vi "Dashboard Main.vi"() -> ()   [LabVIEW 2017]
uses:
  <vilib>/Utility/miscctls.llb/LVRowAndColumnTypeDef.ctl
  <vilib>/event_ctls.llb/eventvkey.ctl
  <vilib>/Rock Robotics/Network Tables/NT Read Numeric Array.vi
  <vilib>/Rock Robotics/Network Tables/NT Read Boolean.vi
  <vilib>/Rock Robotics/WPI/Dashboard/WPI_DashboardLogging Global.vi
panel:
  in  "Camera Settings Right":T1={"Frame Rate"=30, "Compression"=30, "Size"=1, "DB Camera Config"=FALSE} {"Frame Rate" scale=1.0..30.0; "Compression" scale=100.0..-1.0; "Size" items=["640x480", "320x240", "160x120"]}
  in  "Camera Name Right":string(combo)="No Camera Selection"
  out "Camera Info":cluster{"Mbps LED":bool, "Mbps":dbl, "fps":dbl} {"fps" format="%#.1g"; "Mbps" format="%#.1g"}
  in  "Camera Settings":T1={"Frame Rate"=30, "Compression"=30, "Size"=1, "DB Camera Config"=FALSE} {"Frame Rate" scale=1.0..30.0; "Compression" scale=100.0..-1.0; "Size" items=["640x480", "320x240", "160x120"]}
  in  "TCP":refnum<k5>
  in  "Rec Mode":enum32{"Stop", "Record", "Playback"}(radio)
  out "Robot IP":string
  out "Image Message":string="Timeout in Camera Communications"
  in  "Dashboard Tab":T2(tab)
  out "?":bool
  out "?":bool
  out "?":dbl
  in  "Select Auto":string(combo)="Select Autonomous ..."
  out "NT Connection":bool
  out "MotorChart R":cluster{"Numeric":dbl, "Numeric":dbl}(graph)
  out "MotorChart L":cluster{"Numeric":dbl, "Numeric":dbl}(graph)
  out "MotorSliders R":cluster{"MotorSlide1":dbl, "MotorSlide2":dbl} {"MotorSlide2" scale=-1.0..1.0 scale format="%#_2e"; "MotorSlide1" scale=-1.0..1.0 scale format="%#_2e"}
  out "MotorSliders L":cluster{"MotorSlide1":dbl, "MotorSlide2":dbl} {"MotorSlide2" scale=-1.0..1.0 scale format="%#_2e"; "MotorSlide1" scale=-1.0..1.0 scale format="%#_2e"}
  out "Gyro":dbl(knob) scale=0.0..360.0
  out "JS1 Z":dbl(slide) scale=-1.0..1.0 scale format="%#_2e"
  out "JS1 Graph":cluster{"X":dbl, "Y":dbl}[](graph)
  out "JS1 Buttons":T3
  out "JS2 Z":dbl(slide) scale=-1.0..1.0 scale format="%#_2e"
  out "JS2 Graph":cluster{"X":dbl, "Y":dbl}[](graph)
  out "JS2 Buttons":T3
  out "Mode":T4(ring)=enum."Auto Disabled"
  out "Camera Image Right":T5(plugin-control)
  in  "DB/String 9":string
  in  "DB/String 8":string
  in  "DB/String 7":string
  in  "DB/String 6":string
  in  "DB/String 5":string
  in  "DB/String 4":string
  in  "DB/String 3":string
  in  "DB/String 2":string
  in  "DB/String 1":string
  in  "DB/String 0":string
  in  "DB/Slider 0":dbl(slide) scale=0.0..5.0
  in  "DB/Slider 1":dbl(slide) scale=0.0..5.0
  in  "DB/Slider 2":dbl(slide) scale=0.0..5.0
  in  "DB/Slider 3":dbl(slide) scale=0.0..5.0
  out "DB/LED 3":bool
  out "DB/LED 2":bool
  out "DB/LED 1":bool
  out "DB/LED 0":bool
  in  "DB/Button 3":bool
  in  "DB/Button 2":bool
  in  "DB/Button 1":bool
  in  "DB/Button 0":bool caption="New Name"
  in  "Test Slider":dbl(slide) scale=0.0..100.0 scale format="%#_3g"
  in  "On/Off":bool caption="Solenoid"
  in  "Test Name":u16(ring) items=["Select the test to run..."]
  in  "Test Tree":string(tree)
  in  "Motor":cluster{"Value":dbl, "Enable":bool} {"Value" scale=-1.0..1.0 scale format="%#_3g"}
  out "Progress":T6 {"Test Progress" scale=0.0..100.0}
  in  "Rev/Fwd":cluster{"Forward":bool, "Reverse":bool}
  in  "Test Ring":u16(ring) items=["Monochrome", "Color"]
  out "Cmd Status":string
  in  "Execute Command":bool
  in  "Command Params":string[][](table)
  in  "Command Selection":i32(listbox)
  in  "CheckList":i32(listbox)
  out "Tree":string(tree)
  out "Camera Image":T5(plugin-control)
  out "Background":bool
  in  "Camera Name":string(combo)="No Camera Selection"
  # "HW"
  # "HW"
  # "Joysticks"
  # "Ultrasonic Distance"
  # "Drive Motors"
  # "Front"
  # "Limit Switch Position"
  # "Compressor On/Off"
  # "Right"
  # "Left"
  # "Back"
  # "This tab is a great place for autonomous settings and robot-specific values.\nPlace controls and indicators inside this tab and match name to\nDashboard Variables on robot. You can also delete this comment."
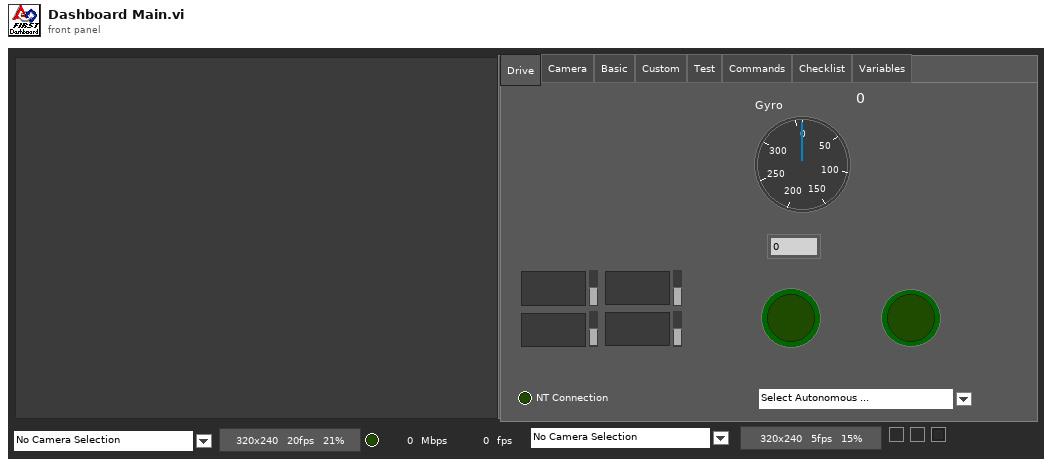
[diagram p1: front panel]
types:
  T1 = cluster{"Frame Rate":i32, "Compression":i32, "Size":u16, "DB Camera Config":bool}
  T2 = enum32{"Drive", "Camera", "Basic", "Custom", "Test", "Commands", "Checklist", "Variables"}
  T3 = cluster{bool, bool, bool, bool, bool, bool, bool, bool, bool, bool, bool, bool}
  T4 = enum8{"Tele-Op Disabled", "Tele-Op Enabled", "Auto Disabled", "Auto Enabled", "Test Disabled", "Test Enabled", "Disconnected", "No Code", "E-Stop"}
  T5 = typedef "IMAQ Image.ctl" = refnum<image>
  T6 = cluster{"Test Progress":u8, "Test Progress Text":string}
  T7 = cluster{"Save Path":path, "Interval (s)":dbl, "Keep":i32}
  T8 = typedef "Image Type" = u32
  T9 = cluster{"IDs":cluster{"RPC field ID":u16, "Unique ID":u16}, "String":string}
  T10 = cluster{"Error Strings":string, "Disable Counts":cluster{u16, u16}, "Rail Faults":cluster{u16, u16, u16}, "Robot IP":string, "DB Mode":u8, "Event Info":cluster{"Name":string, "Type":u8, "Number":u16, "Replay":u8}}
  T11 = cluster{"Storage":cluster{"Disk Free":u64, "RAM Block":u32, "RAM free":u32}, "CPU Utilization":cluster{"CPU % ISR":sgl, "CPU % Time Crit":sgl, "CPU % Timed Str":sgl, "CPU % High":sgl, "CPU % Above":sgl, "CPU % Normal":sgl, "CPU % Low":sgl}, "CAN":cluster{"% Bus Utilization":sgl, "Bus Off Cnt":u32, "TX_FIFO Full Cnt":u32, "Receive Error Cnt":u8, "Transmit Error Cnt":u8}, "HID":cluster{"HID Outputs":u32, "Rumble Low":u16, "Rumble High":u16}[]}
  T12 = cluster{"Status bits":cluster{"Test Mode":bool, "Autonomous":bool, "Enabled":bool, "Code Start":bool, "Brownout":bool, "Reserved 2":bool, "Reserved 3":bool, "E-Stop":bool}, "Code Trace":cluster{"Disabled":bool, "TeleOp":bool, "Auto":bool, "Test":bool}, "Controller Type":enum16{"unknown", "cRIO", "roboRio"}, "Code?":enum16{"unknown", "noCode", "code"}, "Battery V":dbl}
  T13 = cluster{"Control Bits":cluster{"TestMode":bool, "Autonomous":bool, "Enabled":bool, "FMS Present":bool, bool, bool, bool, "E-Stop":bool}, "Team Station ":u8, "Countdown":sgl, "Joystick Values":cluster{"Axes":dbl[], "Buttons":bool[], "POVs":i16[]}[]}
  T14 = cluster{"Axes":dbl[], "Buttons":bool[], "POVs":i16[]}[]
  T15 = cluster{"Axes":dbl[], "Buttons":bool[], "POVs":i16[]}
  T16 = cluster{"Buttons[0]":bool, "Buttons[1]":bool, "Buttons[2]":bool, "Buttons[3]":bool, "Buttons[4]":bool, "Buttons[5]":bool, "Buttons[6]":bool, "Buttons[7]":bool, "Buttons[8]":bool, "Buttons[9]":bool, "Buttons[10]":bool, "Buttons[11]":bool}
  T17 = cluster{"Camera Image":refnum<vi>, "Dashboard Tab":refnum<vi>, "Background":refnum<vi>, "Rec Mode":refnum<vi>, "Test Slider":refnum<vi>, "On/Off ":refnum<vi>, "Test Ring":refnum<vi>, "Rev/Fwd":refnum<vi>, "Test Name":refnum<vi>, "Motor":refnum<vi>, "Progress":refnum<vi>, "CheckList":refnum<vi>, "Tree":refnum<vi>, "Test Tree":refnum<vi>, "Command Params":refnum<vi>, "Command Selection":refnum<vi>, "Execute Command":refnum<vi>, "Cmd Status":refnum<vi>, "Camera Settings":refnum<vi>, "Camera Name":refnum<vi>, "Camera Info":refnum<vi>, "Camera Settings Right":refnum<vi>, "Camera Name Right":refnum<vi>, "Camera Image Right":refnum<vi>}
  T18 = cluster{"Camera Name":string, string, "Saved DB Images Info":cluster{"Save Path":path, "Interval (s)":dbl, "Keep":i32}}
  T19 = cluster{"Camera Name Right":string, string, "Saved DB Images Info":cluster{"Save Path":path, "Interval (s)":dbl, "Keep":i32}}
  T20 = cluster{"Operation":enum16{"Update", "Clear"}, "Color Box":u32}[]
  T21 = typedef "eventvkey.ctl" = enum16{"ASCII", "Enter", "Return", "Shift", "Ctrl", "Alt", "Cmd", "Opt", "Caps", "NumLock", "Clear", "Break", "Up", "Down", "Left", "Right", "Insert", "Delete", "Home", "End", "PageUp", "PageDown", "Escape", "Help", "Pause", "ScrollLock", "F1", "F2", "F3", "F4", "F5", "F6", "F7", "F8", "F9", "F10", "F11", "F12", "F13", "F14", "F15", "F16", "F17", "F18", "F19", "F20", "F21", "F22", "F23", "F24", "Play", "VolumeUp", "VolumeDown", "Mute", "Two Byte Char"}
  T22 = cluster{"Image Size":bool, "Image Type":bool, "Pixel Value":bool, "ROI Information":bool, "Zoom Factor":bool}
  T23 = cluster{"Operation":enum16{"Update", "Clear"}, "Color Box":u32}
  T24 = typedef "LVRowAndColumnTypeDef.ctl" = cluster{"Row":i32, "Column":i32}
  T25 = cluster{"Shift":bool, "Ctrl":bool, "Alt":bool, "Cmd":bool, "Opt":bool}
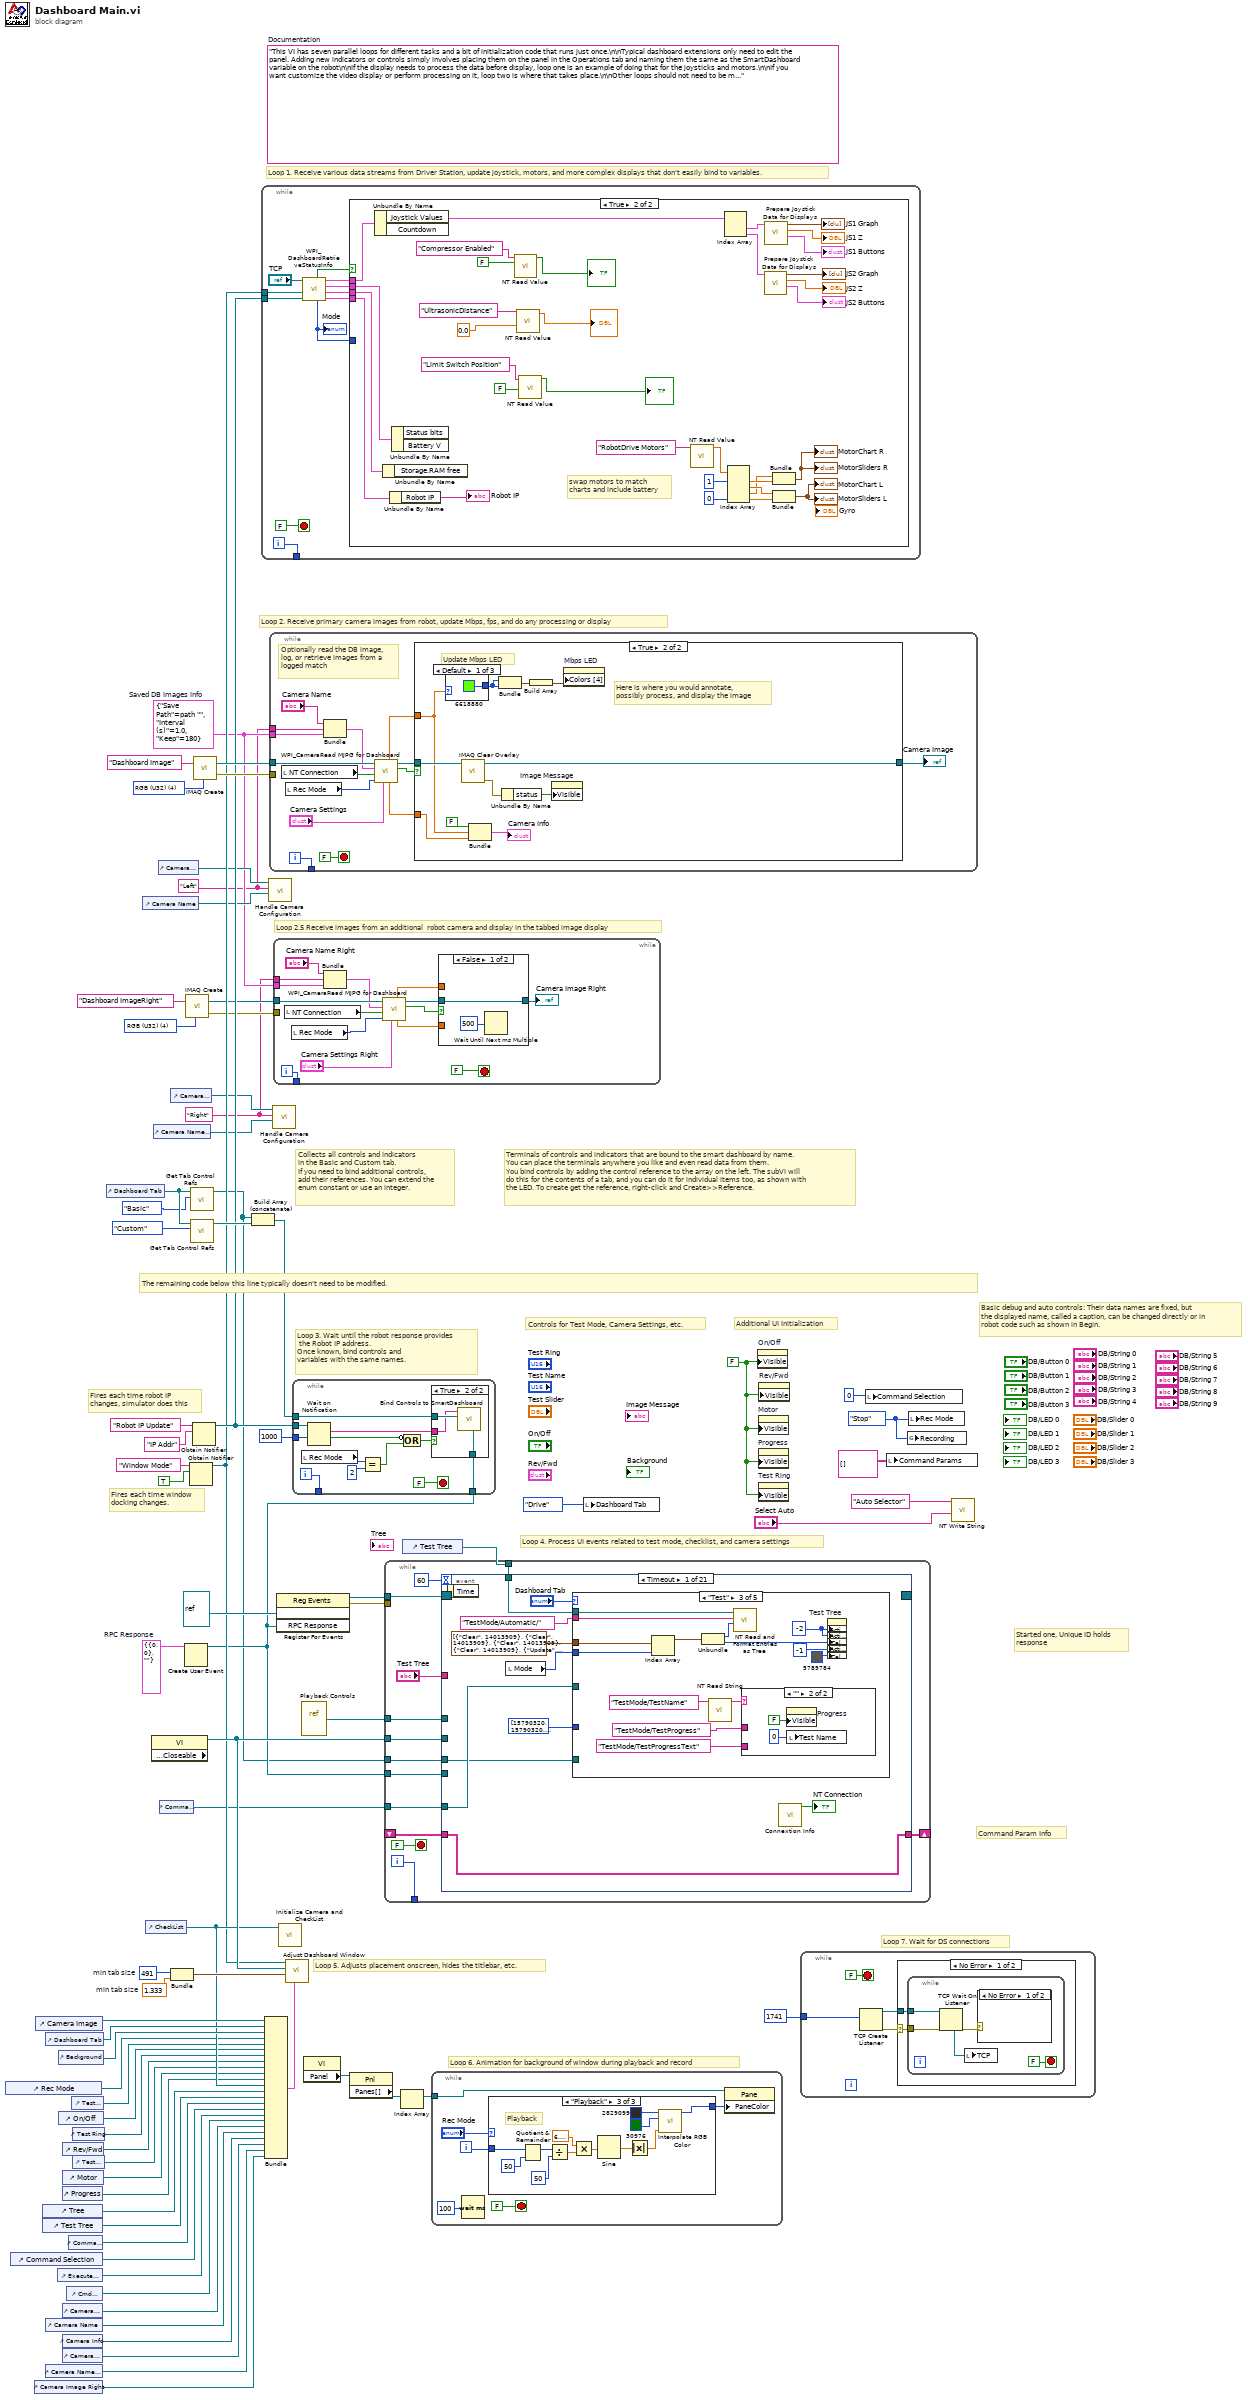
[diagram p0: block diagram]
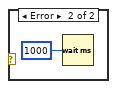
[diagram p3: hidden frame]
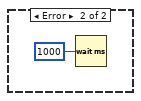
[diagram p4: hidden frame]
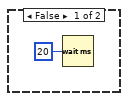
[diagram p5: hidden frame]
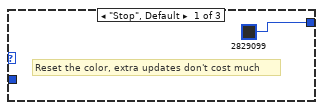
[diagram p6: hidden frame]
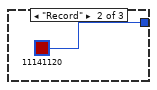
[diagram p7: hidden frame]
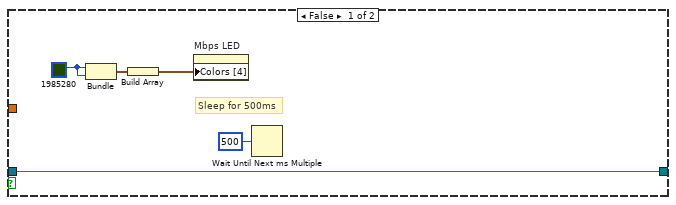
[diagram p9: hidden frame]
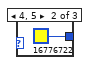
[diagram p10: hidden frame]
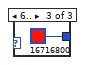
[diagram p11: hidden frame]
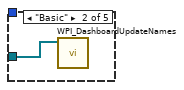
[diagram p13: hidden frame]
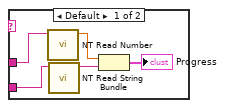
[diagram p14: hidden frame]
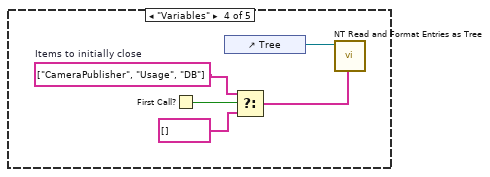
[diagram p15: hidden frame]
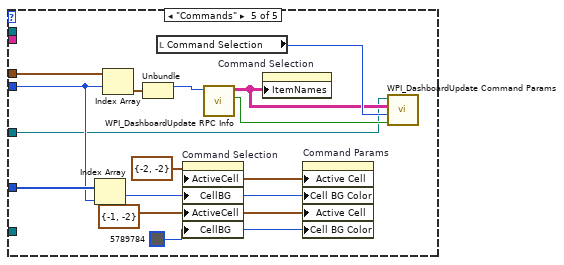
[diagram p16: hidden frame]
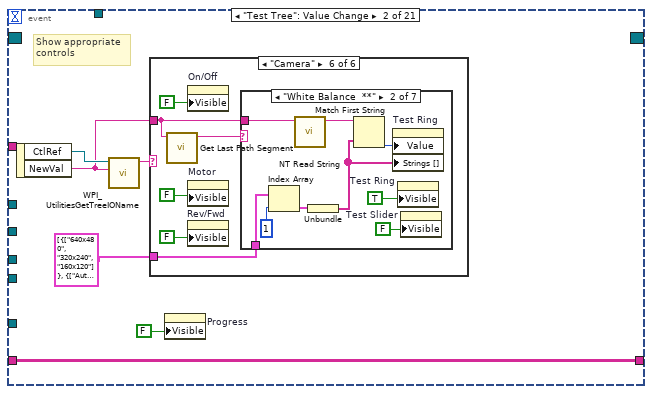
[diagram p17: hidden frame]
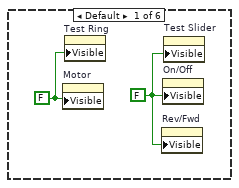
[diagram p18: hidden frame]
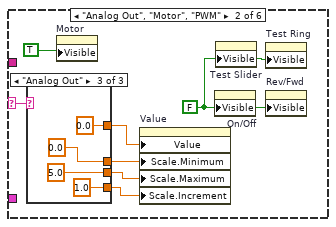
[diagram p19: hidden frame]
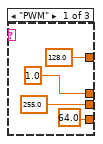
[diagram p20: hidden frame]
diagram:
  w3 = T7 {"Save Path"=path "", "Interval (s)"=1.0, "Keep"=180}  # Saved DB Images Info
  w2 = "Right"
  w1 = "Left"
  w13 = T8 4 items=["Grayscale (U8)", "Grayscale (I16)", "Grayscale (SGL)", "Complex (CSG)", "RGB (U32)", "HSL (U32)", "RGB (U64)"] ("Image Type")
  w29 = T9 {"IDs"={"RPC field ID"=0, "Unique ID"=0}, "String"=""}  # RPC Response
  w52 = 491  # min tab size
  w51 = 1.333  # min tab size
  w59 = enum32{"Stop", "Record", "Playback"}."Stop" ("Rec Mode")
  w36 = FALSE ("Visible")
  (unwired) "This VI has seven parallel loops for different tasks and a bit of initialization code that runs just once.\n\nTypical dashboard extensions only need to edit the panel. Adding new indicators or controls simply involves placing them on the panel in the Operations tab and naming them the same as the SmartDashboard variable on the robot\n\nIf the display needs to process the data before display, loop one is an example of doing that for the joysticks and motors.\n\nIf you want customize the video display or perform processing on it, loop two is where that takes place.\n\nOther loops should not need to be modified. They are pretty standard, and document the task they perform."  # Documentation
  w76 = T8 4 items=["Grayscale (U8)", "Grayscale (I16)", "Grayscale (SGL)", "Complex (CSG)", "RGB (U32)", "HSL (U32)", "RGB (U64)"] ("Image Type")
  # "Loop 2.5 Receive images from an additional  robot camera and display in the tabbed image display"
  # "Command Param Info"
  # "Started one, Unique ID holds\nresponse"
  # "Loop 7. Wait for DS connections"
  # "Basic debug and auto controls: Their data names are fixed, but\nthe displayed name, called a caption, can be changed directly or in\nrobot code such as shown in Begin."
  # "Controls for Test Mode, Camera Settings, etc."
  # "Additional UI Initialization"
  # "Loop 6. Animation for background of window during playback and record"
  # "Fires each time robot IP\nchanges, simulator does this"
  # "Fires each time window\ndocking changes."
  # "Collects all controls and indicators\nin the Basic and Custom tab.\nIf you need to bind additional controls,\nadd their references. You can extend the\nenum constant or use an integer."
  # "The remaining code below this line typically doesn't need to be modified."
  # "Loop 4. Process UI events related to test mode, checklist, and camera settings"
  # "Terminals of controls and indicators that are bound to the smart dashboard by name.\nYou can place the terminals anywhere you like and even read data from them.\nYou bind controls by adding the control reference to the array on the left. The subVI will\ndo this for the contents of a tab, and you can do it for individual items too, as shown with\nthe LED. To create get the reference, right-click and Create>>Reference."
  # "Loop 3. Wait until the robot response provides\n the Robot IP address.\nOnce known, bind controls and\nvariables with the same names."
  # "Loop 5. Adjusts placement onscreen, hides the titlebar, etc."
  # "Loop 1. Receive various data streams from Driver Station, update joystick, motors, and more complex displays that don't easily bind to variables."
  # "Loop 2. Receive primary camera images from robot, update Mbps, fps, and do any processing or display"
  n1 = control-ref of="Rec Mode"() -> (w42:refnum<vi>)
  n2 = control-ref of="Command Selection"() -> (w28:refnum<vi>)
  n3 = control-ref of="Camera Image Right"() -> (w6:refnum<vi>)
  n4 = control-ref of="Camera Image"() -> (w54:refnum<vi>)
  n5 = control-ref of="Tree"() -> (w46:refnum<vi>)
  n6 = control-ref of="Test Tree"() -> (w45:refnum<vi>)
  n7 = control-ref of="Dashboard Tab"() -> (w53:refnum<vi>)
  n8 = control-ref of="Camera Name"() -> (w19:refnum<vi>)
  n9 = control-ref of="Camera Name Right"() -> (w7:refnum<vi>)
  n10 = control-ref of="Execute Command"() -> (w30:refnum<vi>)
  n11 = control-ref of="Background"() -> (w49:refnum<vi>)
  n12 = control-ref of="On/Off"() -> (w40:refnum<vi>)
  n13 = control-ref of="Progress"() -> (w37:refnum<vi>)
  n14 = control-ref of="Camera Settings"() -> (w20:refnum<vi>)
  n15 = control-ref of="Camera Info"() -> (w18:refnum<vi>)
  n16 = control-ref of="Camera Settings Right"() -> (w8:refnum<vi>)
  n17 = control-ref of="Rev/Fwd"() -> (w38:refnum<vi>)
  n18 = control-ref of="Motor"() -> (w43:refnum<vi>)
  n19 = control-ref of="Cmd Status"() -> (w24:refnum<vi>)
  n20 = control-ref of="Command Params"() -> (w31:refnum<vi>)
  n21 = control-ref of="Test Slider"() -> (w41:refnum<vi>)
  n22 = control-ref of="Test Ring"() -> (w39:refnum<vi>)
  n23 = control-ref of="Test Name"() -> (w44:refnum<vi>)
  n24 = control-ref of="Dashboard Tab"() -> (w57:refnum<vi>)
  n25 = control-ref of="Camera Name"() -> (w21:refnum<vi>)
  n26 = control-ref of="CheckList"() -> (w47:refnum<vi>)
  n27 = property class="VI" props=["Front Panel.Closeable"]() -> (reference out=w58:refnum<vi>)  [unwired: 2 in, 2 out]
  n28 = control-ref of="Camera Name Right"() -> (w9:refnum<vi>)
  n29 = control-ref of="Camera Settings"() -> (w22:refnum<vi>)
  n30 = control-ref of="Command Params"() -> (w23:refnum<vi>)
  n31 = control-ref of="Camera Settings Right"() -> (w10:refnum<vi>)
  n32 = Bundle("min tab size"=w52, "min tab size"=w51) -> (w50:cluster{"min tab size":i32, "min tab size":dbl})  [unwired: 1 in]
  n33 = Create User Event(user event datatype=w29) -> (user event=w25:refnum<user-event>)  [unwired: 1 in, 1 out]
  n34 = call "IMAQ Create"("Image Name"="Dashboard ImageRight", "Image Type"=w13) -> ("New Image"=w12:T5, "error out"=w11:errorcluster)  [unwired: 2 in, 1 out]
  n35 = Obtain Notifier(name (unnamed)="Window Mode", notification data type=TRUE) -> (notifier out=w34:refnum<notifier>)  [unwired: 2 in, 2 out]
  n36 = call <vilib>:"Get Tab Control Refs.vi"("Page Index"=T2."Basic" ("Dashboard Tab"), "TabControl in"=w57) -> ("ControlsOnPage"=w17:refnum<vi>[])  [unwired: 9 in]
  n37 = call <vilib>:"Get Tab Control Refs.vi"("Page Index"=T2."Custom" ("Dashboard Tab"), "TabControl in"=w57) -> ("ControlsOnPage"=w56:refnum<vi>[])  [unwired: 9 in]
  n38 = Obtain Notifier(name (unnamed)="Robot IP Update", notification data type="IP Addr" ("name (unnamed)")) -> (notifier out=w35:refnum<notifier>)  [unwired: 2 in, 2 out]
  n39 = call "IMAQ Create"("Image Name"="Dashboard Image", "Image Type"=w76) -> ("New Image"=w74:T5, "error out"=w73:errorcluster)  [unwired: 2 in, 1 out]
  n40 = Build Array (concatenate)(w17, w56) -> (w55:refnum<vi>[])
  n41 = while {
    tunnel: [w86] -> _
    tunnel: w35 -> [w80]
    tunnel: w34 -> [w77]
    i -> [w86]
    stop <- FALSE stop-if-true
    n42 = call <vilib>:"WPI_DashboardRetrieveStatusInfo.vi"("Binding Refnum"=w80, "Window Mode Notifier"=w77, "TCP Cnx"="TCP") -> ("Power and Errors"=w81:T10, "Robot Metrics"=w84:T11, "Status Info"=w85:T12, "Control Info"=w82:T13, "Robot Mode"=w79:T4, "Process?"=w83:bool)  [unwired: 3 in]
    "Mode" <- w79
    n43 = case shown="True" w83 {
      tunnel: w85 -> [_ w121]
      tunnel: w84 -> [_ w120]
      tunnel: w82 -> [_ w119]
      tunnel: w81 -> [_ w118]
      tunnel: w79 -> [_ _]
      frame False {
        n44 = Wait (ms)(milliseconds to wait=u32 20) -> ()  [unwired: 1 out]
      }
      frame True {
        # "swap motors to match\ncharts and include battery"
        n45 = Unbundle By Name(w119) -> ("Joystick Values"=w109:T14)  [unwired: 1 out]
        n46 = Unbundle By Name(w120) -> ()  [unwired: 1 out]
        n47 = Unbundle By Name(w118) -> ("Robot IP"=→"Robot IP":string)
        n48 = Unbundle By Name(w121) -> ()  [unwired: 2 out]
        n49 = call-poly <vilib>:"NT Read Value.vi"("Default Value"=FALSE, "Name"="Compressor Enabled") -> ("Boolean"=→"?":bool)  [unwired: 8 in, 1 out]
        n50 = call-poly <vilib>:"NT Read Value.vi"("Default Value"=0.0, "Name"="UltrasonicDistance") -> ("Numeric"=→"?":dbl)  [unwired: 8 in, 1 out]
        n51 = call-poly <vilib>:"NT Read Value.vi"("Default Value"=FALSE, "Name"="Limit Switch Position") -> ("Boolean"=→"?":bool)  [unwired: 8 in, 1 out]
        n52 = call-poly <vilib>:"NT Read Value.vi"("Name"="RobotDrive Motors") -> ("Numeric Array"=w99:dbl[])  [unwired: 9 in, 1 out]
        n53 = Index Array(array=w109) -> (element #1=w108:T15, element #2=w104:T15)  [unwired: 2 in]
        n54 = Index Array(array=w99, index #1=1, index #4=0) -> (element #1=w113:dbl, element #2=w114:dbl, element #3=w112:dbl, element #4=w117:dbl)  [unwired: 2 in]
        n55 = call "Prepare Joystick Data for Displays.vi"("Joystick Values"=w104) -> ("Buttons"=→"JS2 Buttons":T16, "Z Axis"=→"JS2 Z":dbl, "Cartesian Data"=→"JS2 Graph":cluster{"X axis":dbl, "X axis":dbl}[])  [unwired: 8 in]
        n56 = call "Prepare Joystick Data for Displays.vi"("Joystick Values"=w108) -> ("Buttons"=→"JS1 Buttons":T16, "Z Axis"=→"JS1 Z":dbl, "Cartesian Data"=→"JS1 Graph":cluster{"X axis":dbl, "X axis":dbl}[])  [unwired: 8 in]
        n57 = Bundle("Numeric"=w112, "Numeric"=w113) -> (→"MotorChart R" →"MotorSliders R":cluster{"Numeric":dbl, "Numeric":dbl})  [unwired: 1 in]
        n58 = Bundle("Numeric"=w114, "Numeric"=w117) -> (→"MotorChart L" →"MotorSliders L":cluster{"Numeric":dbl, "Numeric":dbl})  [unwired: 1 in]
      }
    }
  }
  n59 = Bundle("Camera Image"=w54, "Dashboard Tab"=w53, "Background"=w49, "Rec Mode"=w42, "Test Slider"=w41, "On/Off"=w40, "Test Ring"=w39, "Rev/Fwd"=w38, "Test Name"=w44, "Motor"=w43, "Progress"=w37, "CheckList"=w47, "Tree"=w46, "Test Tree"=w45, "Command Params"=w31, "Command Selection"=w28, "Execute Command"=w30, "Cmd Status"=w24, "Camera Settings"=w20, "Camera Name"=w19, "Camera Info"=w18, "Camera Settings Right"=w8, "Camera Name Right"=w7, "Camera Image Right"=w6) -> (w48:T17)  [unwired: 1 in]
  n60 = call "Handle Camera Configuration.vi"("CameraNameRef"=w21, "Display Name"=w1, "ClusterRef"=w22) -> ()  [unwired: 9 in]
  n61 = while {
    tunnel: w74 -> [w134]
    tunnel: w73 -> [_]
    tunnel: [w135] -> _
    tunnel: w3 -> [w125]
    tunnel: w1 -> [w122]
    i -> [w135]
    stop <- FALSE stop-if-true
    # "Optionally read the DB image,\nlog, or retrieve images from a\nlogged match"
    n62 = local read "NT Connection"() -> (w126:bool)
    n63 = local read "Rec Mode"() -> (w130:enum32{"Stop", "Record", "Playback"})
    n64 = Bundle("Camera Name"="Camera Name", w122, "Saved DB Images Info"=w125) -> (w124:T18)  [unwired: 1 in]
    n65 = call <vilib>:"WPI_CameraRead MJPG for Dashboard.vi"("Camera Settings"="Camera Settings", "Rec Mode"=w130, "NT Connection"=w126, "Capture Info"=w124, "Refnum in"=w134) -> ("Active"=w132:bool, "Refnum out"=w133:T5, "FPS"=w131:dbl, "Bandwidth (Mbps)"=w129:dbl)  [unwired: 3 in]
    n66 = case shown="True" w132 {
      tunnel: w133 -> [w137 w148]
      tunnel: w129 -> [_ w145]
      tunnel: w131 -> [_ w146]
      tunnel: [w137 w142] -> w127
      frame False {
        w139 = u32 1985280 ("Color Box")
        # "Sleep for 500ms"
        n67 = Bundle("Color Box"=w139, "Color Box"=w139) -> (w140:cluster{"Color Box":u32, "Color Box":u32})  [unwired: 1 out]
        n68 = Build Array(w140) -> (w138:cluster{"Color Box":u32, "Color Box":u32}[])
        n69 = property on="Mbps LED" class="Bool (strict)"("Colors [4]"=w138) -> ()  [unwired: 2 in, 2 out]
        n70 = Wait Until Next ms Multiple(millisecond multiple=u32 500) -> ()  [unwired: 1 out]
      }
      frame True {
        # "Here is where you would annotate,\npossibly process, and display the image"
        # "Update Mbps LED"
        n71 = case shown="Default" w145 {
          tunnel: [u32 6618880 ("Color Box") u32 16776722 ("Color Box") u32 16716800 ("Color Box")] -> w149
          frame Default {
          }
          frame 4, 5 {
          }
          frame 6.. {
          }
        }
        n72 = call "IMAQ Clear Overlay"("Image"=w148) -> ("error out"=w151:errorcluster, "Image Out"=w142:T5)  [unwired: 2 in, 7 out]
        n73 = Bundle(FALSE, "Bandwidth (Mbps)"=w145, "FPS"=w146) -> (→"Camera Info":cluster{bool, "Bandwidth (Mbps)":dbl, "FPS":dbl})  [unwired: 1 in]
        n74 = Bundle("Color Box"=w149, "Color Box"=w149) -> (w150:cluster{"Color Box":u32, "Color Box":u32})  [unwired: 1 out]
        n75 = Unbundle By Name(w151) -> ("status"=w152:bool)
        n76 = Build Array(w150) -> (w147:cluster{"Color Box":u32, "Color Box":u32}[])
        n77 = property on="Image Message" class="Str"("Visible"=w152) -> ()  [unwired: 2 in, 2 out]
        n78 = property on="Mbps LED" class="Bool (strict)"("Colors [4]"=w147) -> ()  [unwired: 2 in, 2 out]
      }
    }
    "Camera Image" <- w127
  }
  n79 = call "Handle Camera Configuration.vi"("CameraNameRef"=w9, "Display Name"=w2, "ClusterRef"=w10) -> ()  [unwired: 9 in]
  n80 = while {
    tunnel: w12 -> [w170]
    tunnel: w11 -> [_]
    tunnel: [w165] -> _
    tunnel: w3 -> [w159]
    tunnel: w2 -> [w156]
    i -> [w165]
    stop <- FALSE stop-if-true
    n81 = local read "NT Connection"() -> (w160:bool)
    n82 = local read "Rec Mode"() -> (w169:enum32{"Stop", "Record", "Playback"})
    n83 = Bundle("Camera Name Right"="Camera Name Right", w156, "Saved DB Images Info"=w159) -> (w158:T19)  [unwired: 1 in]
    n84 = call <vilib>:"WPI_CameraRead MJPG for Dashboard.vi"("Camera Settings"="Camera Settings Right", "Rec Mode"=w169, "NT Connection"=w160, "Capture Info"=w158, "Refnum in"=w170) -> ("Active"=w164:bool, "Refnum out"=w167:T5, "FPS"=w162:dbl, "Bandwidth (Mbps)"=w163:dbl)  [unwired: 3 in]
    n85 = case shown="False" w164 {
      tunnel: w167 -> [w171 w173]
      tunnel: w163 -> [_ _]
      tunnel: w162 -> [_ _]
      tunnel: [w171 w173] -> w161
      frame False {
        n86 = Wait Until Next ms Multiple(millisecond multiple=u32 500) -> ()  [unwired: 1 out]
      }
      frame True {
      }
    }
    "Camera Image Right" <- w161
  }
  n87 = register-events(refnum<vi> refnum, w25) -> (reference out=w63:refnum<event-registration>, error out=w62:errorcluster)  [unwired: 2 in]
  n88 = call "Initialize Camera and CheckList.vi"("ListBox in"=w47) -> ()  [unwired: 11 in]
  n89 = call "Adjust Dashboard Window.vi"("Sizing Refnums"=w48, "Size Constraints"=w50, "VI"=w58, "WIn Mode"=w34) -> ()  [unwired: 8 in]
  n90 = while {
    tunnel: w55 -> [w185]
    tunnel: w35 -> [w183]
    tunnel: [w181] -> _
    tunnel: u32 1000 ("milliseconds to wait") -> [w180]
    tunnel: w25 -> [w174]
    i -> [w181]
    stop <- FALSE stop-if-true
    n91 = local read "Rec Mode"() -> (w176:enum32{"Stop", "Record", "Playback"})
    n92 = Wait on Notification(notifier=w183, timeout in ms (-1)=w180) -> (notification=w182:string, timed out?=w178:bool)  [unwired: 2 in, 2 out]
    n93 = Equal?(x=w176, y=u16 2 ("Rec Mode")) -> (x = y?=w177:bool)
    n94 = Compound Arithmetic op=OR(invert w178, w177) -> (w179:bool)
    n95 = case shown="True" w179 {
      tunnel: w185 -> [_ w188]
      tunnel: w182 -> [_ w187]
      tunnel: w174 -> [_ w186]
      frame False {
      }
      frame True {
        n96 = call <vilib>:"Bind Controls to SmartDashboard.vi"("RPC ref"=w186, "Bound Control Refs"=w188, "Server IP Address"=w187) -> ()  [unwired: 9 in]
      }
    }
  }
  n97 = vi-ref "Playback Controls.vi"() -> (w64:refnum<vi>)
  n98 = property class="VI"() -> ("Panel"=w66:refnum<vi>)  [unwired: 2 in, 2 out]
  n99 = property class="Pnl"(reference=w66) -> ("Panes[]"=w67:refnum<vi>[])  [unwired: 1 in, 2 out]
  n100 = Index Array(array=w67) -> (element=w65:refnum<vi>)  [unwired: 1 in]
  n101 = control-ref of="Test Tree"() -> (w68:refnum<vi>)
  n102 = while {
    tunnel: [w198] -> _
    tunnel: w68 -> [w197]
    tunnel: w64 -> [w196]
    tunnel: w63 -> [w195]
    tunnel: w62 -> [_]
    tunnel: w58 -> [w194]
    tunnel: w25 -> [w193]
    tunnel: w23 -> [w192]
    shift-right: [w191] -> _
    shift-left: _ -> [w190]
    tunnel: w17 -> [w189]
    i -> [w198]
    stop <- FALSE stop-if-true
    n103 = event shown="[0] Timeout" {
      selector: w195 -> [_ _ _ _ _ _ _ _ _ _ _ _ _ _ _ _ _ _ _ _ _]
      dyn-events: [_ _ _ _ _ _ _ _ _ _ _ _ _ _ _ _ w458 _ _ _ _] -> _
      timeout: u32 60 ("milliseconds to wait") -> [_ _ _ _ _ _ _ _ _ _ _ _ _ _ _ _ _ _ _ _ _]
      tunnel: w197 -> [w210 _ _ _ _ _ _ _ _ _ _ _ _ _ _ _ _ _ _ _ _]
      tunnel: "Test Tree" -> [_ _ _ _ _ _ _ _ _ _ _ w425 w433 w435 w439 w447 _ _ _ _ _]
      tunnel: w196 -> [_ _ _ _ _ _ _ _ _ _ _ _ _ _ _ _ w460 _ w478 _ _]
      tunnel: w194 -> [_ _ _ _ _ _ _ _ _ _ _ _ _ _ _ _ w456 _ _ _ _]
      tunnel: w193 -> [_ _ _ _ _ _ _ _ _ _ _ _ _ _ _ _ w454 _ _ _ _]
      tunnel: w192 -> [w205 _ _ _ _ _ w376 _ _ _ _ _ _ _ _ _ _ _ _ _ _]
      tunnel: [w204 w253 w355 w360 w369 w373 w374 w383 w393 w400 w412 w424 w431 w434 w438 w446 w453 w473 w475 w479 w492] -> w191
      tunnel: w190 -> [w204 w253 w355 w360 w369 w373 w374 _ _ w400 w412 w424 w431 w434 w438 w446 w453 w473 w475 w479 w492]
      tunnel: w189 -> [w202 _ _ _ _ _ _ _ _ _ _ _ _ _ _ _ _ _ _ _ _]
      event Timeout {
        n104 = event-data() -> ()  [unwired: 1 in, 1 out]
        n105 = local read "Mode"() -> (w207:T4)
        n106 = case shown="\"Test\"" "Dashboard Tab" {
          tunnel: w210 -> [_ _ w226 _ _]
          tunnel: "TestMode/Automatic/" ("Name Pattern") -> [_ _ w225 _ _]
          tunnel: T20 [{"Operation"=enum."Clear", "Color Box"=14013909}, {"Operation"=enum."Clear", "Color Box"=14013909}, {"Operation"=enum."Clear", "Color Box"=14013909}, {"Operation"=enum."Clear", "Color Box"=14013909}, {"Operation"=enum."Update", "Color Box"=14013909}, {"Operation"=enum."Update", "Color Box"=16777215}, {"Operation"=enum."Clear", "Color Box"=14013909}, {"Operation"=enum."Clear", "Color Box"=14013909}, {"Operation"=enum."Clear", "Color Box"=14013909}] -> [_ _ w218 _ w246]
          tunnel: w207 -> [_ _ w217 _ w245]
          tunnel: u32[] [15790320, 15790320, 15790320, 15790320, 16777215, 16777215, 15790320, 15790320, 15790320] -> [_ _ _ _ w251]
          tunnel: w205 -> [_ _ _ _ w239]
          tunnel: w202 -> [_ w212 _ _ _]
          frame "Custom", Default {
          }
          frame "Basic" {
            n107 = call <vilib>:"WPI_DashboardUpdateNames.vi"("Controls on Tab"=w212) -> ()  [unwired: 11 in]
          }
          frame "Test" {
            w224 = -2 ("Active Item:Row Number")
            n108 = Index Array(array=w218, index=w217) -> (element=w219:T23)
            n109 = Unbundle(w219) -> ("Operation"=w220:enum16{"Update", "Clear"}, "Color Box"=w221:u32)
            n110 = call <vilib>:"NT Read String.vi"("Name"="TestMode/TestName") -> ("String"=w215:string)  [unwired: 9 in, 1 out]
            n111 = call <vilib>:"NT Read and Format Entries as Tree.vi"("Operation"=w220, "Name Pattern"=w225, "Tree Refnum"=w226) -> ()  [unwired: 7 in, 2 out]
            n112 = case shown="\"\"" w215 {
              tunnel: "TestMode/TestProgress" ("Name") -> [w228 _]
              tunnel: "TestMode/TestProgressText" ("Name") -> [w227 _]
              frame Default {
                n113 = call <vilib>:"NT Read Number.vi"("Name"=w228) -> ("Numeric"=w229:dbl)  [unwired: 9 in, 1 out]
                n114 = call <vilib>:"NT Read String.vi"("Name"=w227) -> ("String"=w230:string)  [unwired: 9 in, 1 out]
                n115 = Bundle("Numeric"=w229, "String"=w230) -> (→"Progress":cluster{"Numeric":dbl, "String":string})  [unwired: 1 in]
              }
              frame "" {
                n116 = property on="Progress" class="Clust (strict)"("Visible"=FALSE) -> ()  [unwired: 2 in, 2 out]
                n117 = local write "Test Name"(u16 0) -> ()
              }
            }
            n118 = property on="Test Tree" class="Tree (strict)"("Active Item Row Number"=w224, "ActiveColNum"=w224, "CellBG"=w221, "Active Item Row Number"=-1 ("Active Item:Row Number"), "CellBG"=u32 5789784 ("Color Box")) -> ()  [unwired: 2 in, 2 out]
          }
          frame "Variables" {
            w236 = string[] ["CameraPublisher", "Usage", "DB"]  # Items to initially close
            n119 = First Call?() -> (First Call?: T/F=w237:bool)
            n120 = control-ref of="Tree"() -> (w238:refnum<vi>)
            n121 = Select(t=w236, s=w237, f=string[] []) -> (s? t:f=w234:string[])
            n122 = call <vilib>:"NT Read and Format Entries as Tree.vi"("Tags to  Close"=w234, "Tree Refnum"=w238) -> ()  [unwired: 8 in, 2 out]
          }
          frame "Commands" {
            w247 = u32 5789784 ("Color Box")
            w248 = T24 {"Row"=-1, "Column"=-2} ("Active Cell:Active Cell")
            w250 = T24 {"Row"=-2, "Column"=-2} ("Active Cell:Active Cell")
            n123 = Index Array(array=w251, index=w245) -> (element=w249:u32)
            n124 = Index Array(array=w246, index=w245) -> (element=w244:T23)
            n125 = Unbundle(w244) -> ("Operation"=w243:enum16{"Update", "Clear"})  [unwired: 1 out]
            n126 = local read "Command Selection"() -> (w242:i32)
            n127 = property on="Command Selection" class="MCListbox (strict)"("ActiveCell"=w250, "CellBG"=w249, "ActiveCell"=w248, "CellBG"=w247) -> ()  [unwired: 2 in, 2 out]
            n128 = call <vilib>:"WPI_DashboardUpdate RPC Info.vi"("Operation"=w243) -> ("update"=w241:bool, "commands"=w240:string[][])  [unwired: 9 in]
            n129 = property on="Command Selection" class="MCListbox (strict)"("ItemNames"=w240) -> ()  [unwired: 2 in, 2 out]
            n130 = property on="Command Params" class="Tbl (strict)"("Active Cell"=w250, "Cell BG Color"=w249, "Active Cell"=w248, "Cell BG Color"=w247) -> ()  [unwired: 2 in, 2 out]
            n131 = call <vilib>:"WPI_DashboardUpdate Command Params.vi"("Update"=w241, "NewVal"=w242, "Commands"=w240, "Param Tbl"=w239) -> ()  [unwired: 7 in, 1 out]
          }
        }
        n132 = call <vilib>:"Connextion Info.vi"() -> ("Connected"=→"NT Connection":bool)  [unwired: 10 in, 1 out]
      }
      event "Test Tree": Value Change {
        # "Show appropriate\ncontrols"
        n133 = event-data() -> ("CtlRef"=w256:refnum<vi>, "NewVal"=w254:string)  [unwired: 1 in]
        n134 = call <vilib>:"WPI_UtilitiesGetTreeIOName.vi"("NewVal"=w254, "TreeControl in"=w256) -> ("I/O Name"=w257:string)  [unwired: 9 in]
        n135 = case shown="\"Camera\"" w257 {
          selector: w257 -> [_ w264 _ w286 w295 _]
          tunnel: w254 -> [_ _ w283 w285 _ w302]
          tunnel: cluster{string[]}[] [{["640x480", "320x240", "160x120"]}, {["Auto", "Fixed indoor", "Fixed outdoor 1", "Fixed outdoor 2", "Fixed fluorescent 1", "Fixed fluorescent 2", "Hold current"]}, {["Auto", "Flicker-free 50 Hz", "Flicker-free 60 Hz", "Hold current"]}, {["None", "Prioritize frame rate", "Prioritize image quality"]}, {["Monochrome", "Color"]}] -> [_ _ _ _ _ w301]
          frame Default {
            w259 = FALSE ("Visible")
            w258 = FALSE ("Visible")
            n136 = property on="Motor" class="Clust (strict)"("Visible"=w258) -> ()  [unwired: 2 in, 2 out]
            n137 = property on="Test Ring" class="Ring (strict)"("Visible"=w258) -> ()  [unwired: 2 in, 2 out]
            n138 = property on="Rev/Fwd" class="Clust (strict)"("Visible"=w259) -> ()  [unwired: 2 in, 2 out]
            n139 = property on="On/Off" class="Bool (strict)"("Visible"=w259) -> ()  [unwired: 2 in, 2 out]
            n140 = property on="Test Slider" class="Slide (strict)"("Visible"=w259) -> ()  [unwired: 2 in, 2 out]
          }
          frame "Analog Out", "Motor", "PWM" {
            w265 = FALSE ("Visible")
            n141 = case shown="\"Analog Out\"" w264 {
              tunnel: [1.0 ("Value") -1.0 ("Value") 0.0 ("Value")] -> w263
              tunnel: [255.0 ("Value") 1.0 ("Value") 5.0 ("Value")] -> w262
              tunnel: [128.0 ("Value") 0.0 ("Value") 0.0 ("Value")] -> w261
              tunnel: [64.0 ("Value") 0.5 ("Value") 1.0 ("Value")] -> w260
              frame "PWM" {
              }
              frame "Motor", Default {
              }
              frame "Analog Out" {
              }
            }
            n142 = property on="Motor" class="Clust (strict)"("Visible"=TRUE) -> ()  [unwired: 2 in, 2 out]
            n143 = property on="Value" class="Slide (strict)"("Value"=w261, "Scale.Minimum"=w263, "Scale.Maximum"=w262, "Scale.Increment"=w260) -> ()  [unwired: 2 in, 2 out]
            n144 = property on="On/Off" class="Bool (strict)"("Visible"=w265) -> ()  [unwired: 2 in, 2 out]
            n145 = property on="Test Slider" class="Slide (strict)"("Visible"=w265) -> ()  [unwired: 2 in, 2 out]
            n146 = property on="Test Ring" class="Ring (strict)"("Visible"=w265) -> ()  [unwired: 2 in, 2 out]
            n147 = property on="Rev/Fwd" class="Clust (strict)"("Visible"=w265) -> ()  [unwired: 2 in, 2 out]
          }
          frame "Servo" {
            w281 = FALSE ("Visible")
            n148 = call <vilib>:"NT Read Number.vi"("Name"=w283) -> ("Numeric"=w282:dbl)  [unwired: 9 in, 1 out]
            n149 = property on="Test Slider" class="Slide (strict)"("Visible"=TRUE, "Scale.Maximum"=170.0 ("Scale.Range:Maximum")) -> ()  [unwired: 2 in, 2 out]
            n150 = local write "Test Slider"(w282) -> ()
            n151 = property on="Motor" class="Clust (strict)"("Visible"=w281) -> ()  [unwired: 2 in, 2 out]
            n152 = property on="Rev/Fwd" class="Clust (strict)"("Visible"=w281) -> ()  [unwired: 2 in, 2 out]
            n153 = property on="On/Off" class="Bool (strict)"("Visible"=w281) -> ()  [unwired: 2 in, 2 out]
            n154 = property on="Test Ring" class="Ring (strict)"("Visible"=w281) -> ()  [unwired: 2 in, 2 out]
          }
          frame "Relay", "Solenoid" {
            w284 = FALSE ("Visible")
            n155 = property on="Motor" class="Clust (strict)"("Visible"=w284) -> ()  [unwired: 2 in, 2 out]
            n156 = property on="Test Slider" class="Slide (strict)"("Visible"=w284) -> ()  [unwired: 2 in, 2 out]
            n157 = Search and Replace String(input string=w285, search string="/Value  **", replace string="/Direction") -> (result string=w291:string)  [unwired: 5 in, 3 out]
            n158 = property on="Test Ring" class="Ring (strict)"("Visible"=w284) -> ()  [unwired: 2 in, 2 out]
            n159 = call <vilib>:"NT Read String.vi"("Name"=w291) -> ("String"=w289:string)  [unwired: 9 in, 1 out]
            n160 = Equal?(x="Both directions", y=w289) -> (x = y?=w287:bool)
            n161 = Not(x=w287) -> (.not. x?=w288:bool)
            n162 = property on="Rev/Fwd" class="Clust (strict)"("Visible"=w287) -> ()  [unwired: 2 in, 2 out]
            n163 = property on="On/Off" class="Bool (strict)"("Visible"=w288, "Caption.Text"=w286) -> ()  [unwired: 2 in, 2 out]
          }
          frame "Compressor", "Digital Out" {
            w294 = FALSE ("Visible")
            # "Get direction and finish"
            n164 = property on="Motor" class="Clust (strict)"("Visible"=w294) -> ()  [unwired: 2 in, 2 out]
            n165 = property on="Test Slider" class="Slide (strict)"("Visible"=w294) -> ()  [unwired: 2 in, 2 out]
            n166 = property on="Test Ring" class="Ring (strict)"("Visible"=w294) -> ()  [unwired: 2 in, 2 out]
            n167 = property on="On/Off" class="Bool (strict)"("Visible"=TRUE, "Caption.Text"=w295) -> ()  [unwired: 2 in, 2 out]
            n168 = property on="Rev/Fwd" class="Clust (strict)"("Visible"=FALSE) -> ()  [unwired: 2 in, 2 out]
          }
          frame "Camera" {
            n169 = call <vilib>:"Get Last Path Segment.vi"("String in"=w302) -> ("String out"=w303:string)  [unwired: 10 in]
            n170 = property on="On/Off" class="Bool (strict)"("Visible"=FALSE) -> ()  [unwired: 2 in, 2 out]
            n171 = property on="Motor" class="Clust (strict)"("Visible"=FALSE) -> ()  [unwired: 2 in, 2 out]
            n172 = property on="Rev/Fwd" class="Clust (strict)"("Visible"=FALSE) -> ()  [unwired: 2 in, 2 out]
            n173 = case shown="\"White Balance  **\"" w303 {
              tunnel: w302 -> [w309 w318 w327 w336 w345 _ w351]
              tunnel: w301 -> [w307 w315 w324 w333 w342 _ _]
              frame "Size  **" {
                n174 = Index Array(array=w307) -> (element=w306:cluster{string[]})  [unwired: 1 in]
                n175 = call <vilib>:"NT Read String.vi"("Name"=w309) -> ("String"=w308:string)  [unwired: 9 in, 1 out]
                n176 = Unbundle(w306) -> (w304:string[])
                n177 = Match First String(2:w304, 3:w308) -> (0:w305:i32)  [unwired: 1 out]
                n178 = property on="Test Ring" class="Ring (strict)"("Value"=w305, "Strings []"=w304) -> ()  [unwired: 2 in, 2 out]
                n179 = property on="Test Ring" class="Ring (strict)"("Visible"=TRUE) -> ()  [unwired: 2 in, 2 out]
                n180 = property on="Test Slider" class="Slide (strict)"("Visible"=FALSE) -> ()  [unwired: 2 in, 2 out]
              }
              frame "White Balance  **" {
                n181 = Index Array(array=w315, index=1) -> (element=w316:cluster{string[]})
                n182 = call <vilib>:"NT Read String.vi"("Name"=w318) -> ("String"=w317:string)  [unwired: 9 in, 1 out]
                n183 = Unbundle(w316) -> (w313:string[])
                n184 = Match First String(2:w313, 3:w317) -> (0:w312:i32)  [unwired: 1 out]
                n185 = property on="Test Ring" class="Ring (strict)"("Value"=w312, "Strings []"=w313) -> ()  [unwired: 2 in, 2 out]
                n186 = property on="Test Ring" class="Ring (strict)"("Visible"=TRUE) -> ()  [unwired: 2 in, 2 out]
                n187 = property on="Test Slider" class="Slide (strict)"("Visible"=FALSE) -> ()  [unwired: 2 in, 2 out]
              }
              frame "Exposure  **" {
                n188 = Index Array(array=w324, index=2) -> (element=w325:cluster{string[]})
                n189 = call <vilib>:"NT Read String.vi"("Name"=w327) -> ("String"=w326:string)  [unwired: 9 in, 1 out]
                n190 = Unbundle(w325) -> (w321:string[])
                n191 = Match First String(2:w321, 3:w326) -> (0:w322:i32)  [unwired: 1 out]
                n192 = property on="Test Ring" class="Ring (strict)"("Value"=w322, "Strings []"=w321) -> ()  [unwired: 2 in, 2 out]
                n193 = property on="Test Ring" class="Ring (strict)"("Visible"=TRUE) -> ()  [unwired: 2 in, 2 out]
                n194 = property on="Test Slider" class="Slide (strict)"("Visible"=FALSE) -> ()  [unwired: 2 in, 2 out]
              }
              frame "Exposure Priority  **" {
                n195 = Index Array(array=w333, index=3) -> (element=w334:cluster{string[]})
                n196 = call <vilib>:"NT Read String.vi"("Name"=w336) -> ("String"=w335:string)  [unwired: 9 in, 1 out]
                n197 = Unbundle(w334) -> (w330:string[])
                n198 = Match First String(2:w330, 3:w335) -> (0:w331:i32)  [unwired: 1 out]
                n199 = property on="Test Ring" class="Ring (strict)"("Value"=w331, "Strings []"=w330) -> ()  [unwired: 2 in, 2 out]
                n200 = property on="Test Ring" class="Ring (strict)"("Visible"=TRUE) -> ()  [unwired: 2 in, 2 out]
                n201 = property on="Test Slider" class="Slide (strict)"("Visible"=FALSE) -> ()  [unwired: 2 in, 2 out]
              }
              frame "Color Enable  **" {
                n202 = Index Array(array=w342, index=4) -> (element=w343:cluster{string[]})
                n203 = call <vilib>:"NT Read String.vi"("Name"=w345) -> ("String"=w344:string)  [unwired: 9 in, 1 out]
                n204 = Unbundle(w343) -> (w339:string[])
                n205 = Match First String(2:w339, 3:w344) -> (0:w340:i32)  [unwired: 1 out]
                n206 = property on="Test Ring" class="Ring (strict)"("Value"=w340, "Strings []"=w339) -> ()  [unwired: 2 in, 2 out]
                n207 = property on="Test Ring" class="Ring (strict)"("Visible"=TRUE) -> ()  [unwired: 2 in, 2 out]
                n208 = property on="Test Slider" class="Slide (strict)"("Visible"=FALSE) -> ()  [unwired: 2 in, 2 out]
              }
              frame Default {
                n209 = property on="Test Ring" class="Ring (strict)"("Visible"=FALSE) -> ()  [unwired: 2 in, 2 out]
                n210 = property on="Test Slider" class="Slide (strict)"("Visible"=FALSE) -> ()  [unwired: 2 in, 2 out]
              }
              frame "Brightness  **", "Color Level  **", "Compression  **", "FPS  **", "Sharpness  **" {
                n211 = call <vilib>:"NT Read Number.vi"("Name"=w351) -> ("Numeric"=w350:dbl)  [unwired: 9 in, 1 out]
                n212 = local write "Test Slider"(w350) -> ()
                n213 = property on="Test Slider" class="Slide (strict)"("Visible"=TRUE, "Scale.Maximum"=100.0 ("Scale.Range:Maximum")) -> ()  [unwired: 2 in, 2 out]
                n214 = property on="Test Ring" class="Ring (strict)"("Visible"=FALSE) -> ()  [unwired: 2 in, 2 out]
              }
            }
          }
        }
        n215 = property on="Progress" class="Clust (strict)"("Visible"=FALSE) -> ()  [unwired: 2 in, 2 out]
      }
      event "Test Name": Mouse Enter {
        # "Populate the ring with the list of tests"
        n216 = event-data() -> ()  [unwired: 1 in, 1 out]
        n217 = call <vilib>:"NT Read String Array.vi"("Name"="TestMode/TestList") -> ("String Array"=w359:string[])  [unwired: 9 in, 1 out]
        n218 = Build Array (concatenate)("Select the test to run...", w359) -> (w358:string[])
        n219 = property on="Test Name" class="Ring (strict)"("Strings []"=w358) -> ()  [unwired: 2 in, 2 out]
      }
      event "Test Name": Value Change {
        w361 = FALSE ("Visible")
        # "Tell the robot the test name to run"
        n220 = event-data() -> ("NewVal"=w365:u16)  [unwired: 1 in]
        n221 = property on="Test Name" class="Ring (strict)"() -> ("Strings []"=w366:string[])  [unwired: 2 in, 2 out]
        n222 = local write "Progress"(T6 {"Test Progress"=0, "Test Progress Text"=""} ("Progress")) -> ()
        n223 = Index Array(array=w366, index=w365) -> (element=w364:string)
        n224 = call <vilib>:"NT Write String.vi"("String"=w364, "Name"="TestMode/TestName") -> ()  [unwired: 9 in, 1 out]
        n225 = property on="Progress" class="Clust (strict)"("Visible"=TRUE) -> ()  [unwired: 2 in, 2 out]
        n226 = property on="Motor" class="Clust (strict)"("Visible"=w361) -> ()  [unwired: 2 in, 2 out]
        n227 = property on="Test Slider" class="Slide (strict)"("Visible"=w361) -> ()  [unwired: 2 in, 2 out]
        n228 = property on="On/Off" class="Bool (strict)"("Visible"=w361) -> ()  [unwired: 2 in, 2 out]
        n229 = property on="Rev/Fwd" class="Clust (strict)"("Visible"=w361) -> ()  [unwired: 2 in, 2 out]
        n230 = property on="Test Ring" class="Ring (strict)"("Visible"=w361) -> ()  [unwired: 2 in, 2 out]
      }
      event "Select Auto": Mouse Enter {
        # "Populate the combo box with the list of autonomous options"
        n231 = event-data() -> ()  [unwired: 1 in, 1 out]
        n232 = call <vilib>:"NT Read String Array.vi"("Name"="Auto List") -> ("String Array"=w368:string[])  [unwired: 9 in, 1 out]
        n233 = property on="Select Auto" class="CmbBox"("Strings[]"=w368) -> ()  [unwired: 2 in, 2 out]
      }
      event "Select Auto": Value Change {
        # "User modified the Auto Selection. Write to NT variable so robot knows."
        n234 = event-data() -> ("NewVal"=w371:string)  [unwired: 1 in]
        n235 = call <vilib>:"NT Write String.vi"("String"=w371, "Name"="Auto Selector") -> ()  [unwired: 9 in, 1 out]
      }
      event "Command Selection": Value Change {
        # "Get the params and show in table"
        n236 = event-data() -> ("NewVal"=w377:i32)  [unwired: 1 in]
        n237 = property on="Command Selection" class="MCListbox (strict)"() -> ("ItemNames"=w375:string[][])  [unwired: 2 in, 2 out]
        n238 = call <vilib>:"WPI_DashboardUpdate Command Params.vi"("NewVal"=w377, "Commands"=w375, "Param Tbl"=w376) -> ()  [unwired: 8 in, 1 out]
      }
      event "Execute Command": Value Change {
        # "Started one, Unique ID holds\nresponse"
        n239 = event-data() -> ()  [unwired: 1 in, 1 out]
        n240 = property on="Command Selection" class="MCListbox (strict)"() -> ("ItemNames"=w388:string[][])  [unwired: 2 in, 2 out]
        n241 = Index Array(array=w388, index (row)="Command Selection", index (col)=0) -> (element=w386:string)
        n242 = call <vilib>:"Invoke Commands.vi"("Command Params"="Command Params", "Function Name"=w386) -> ("Params"=w382:u8, "Started"=w381:bool)  [unwired: 7 in, 1 out]
        n243 = Array Subset(array="Command Params", length (row)=w382) -> (w383:string[][])  [unwired: 3 in]
        n244 = Select(t="Executing" ("Cmd Status"), s=w381, f="" ("Cmd Status")) -> (s? t:f=→"Cmd Status":string)
      }
      event "Command Selection": Double Click {
        n245 = event-data() -> ("Row"=w396:i32)  [unwired: 1 in]
        n246 = property on="Command Selection" class="MCListbox (strict)"() -> ("ItemNames"=w399:string[][])  [unwired: 2 in, 2 out]
        n247 = local read "Command Params"() -> (w395:string[][])
        n248 = Index Array(array=w399, index (row)=w396, index (col)=0) -> (element=w397:string)
        n249 = call <vilib>:"Invoke Commands.vi"("Command Params"=w395, "Function Name"=w397) -> ("Params"=w394:u8, "Started"=w389:bool)  [unwired: 7 in, 1 out]
        n250 = Array Subset(array=w395, length (row)=w394) -> (w393:string[][])  [unwired: 3 in]
        n251 = Select(t="Executing" ("Cmd Status"), s=w389, f="" ("Cmd Status")) -> (s? t:f=w390:string)
        n252 = local write "Cmd Status"(w390) -> ()
      }
      event "CheckList": Double Click {
        # "Shift clears all"
        # "Update symbols on the listbox"
        n253 = event-data() -> ("PlatMods.Shift"=w401:bool, "Row"=w403:i32)  [unwired: 1 in]
        n254 = case shown="True" w401 {
          tunnel: w403 -> [w407 _]
          tunnel: 1 -> [w406 _]
          frame False {
            n255 = property on="CheckList" class="LstBox (strict)"() -> ("Item Symbols"=w405:i32[])  [unwired: 2 in, 2 out]
            n256 = Replace Array Subset(array=w405, new element=w406, index=w407) -> (w404:i32[])
            n257 = property on="CheckList" class="LstBox (strict)"("Item Symbols"=w404) -> ()  [unwired: 2 in, 2 out]
          }
          frame True {
            w408 = 0 ("Top Row")
            n258 = property on="CheckList" class="LstBox (strict)"() -> ("Number of Rows"=w410:u32)  [unwired: 2 in, 2 out]
            n259 = Initialize Array(0, w410) -> (w409:i32[])
            n260 = property on="CheckList" class="LstBox (strict)"("Top Row"=w408, "Value"=w408, "Item Symbols"=w409) -> ()  [unwired: 2 in, 2 out]
          }
        }
      }
      event "CheckList": Key Down {
        # "Update symbols on the listbox\nLeft and right keys check and uncheck"
        n261 = event-data() -> ("VKey"=w414:T21)  [unwired: 1 in]
        n262 = case shown="\"Left\", \"Right\"" w414 {
          selector: w414 -> [w419 _]
          tunnel: eventvkey."Left" ("VKey") -> [w417 _]
          frame "Left", "Right" {
            n263 = Equal?(x=w417, y=w419) -> (x = y?=w418:bool)
            n264 = Select(t=0, s=w418, f=1) -> (s? t:f=w420:i32)
            n265 = property on="CheckList" class="LstBox (strict)"() -> ("Item Symbols"=w423:i32[])  [unwired: 2 in, 2 out]
            n266 = Replace Array Subset(array=w423, new element=w420, index="CheckList") -> (w422:i32[])
            n267 = property on="CheckList" class="LstBox (strict)"("Item Symbols"=w422) -> ()  [unwired: 2 in, 2 out]
          }
          frame Default {
          }
        }
      }
      event "Motor.Enable": Value Change {
        # "When the test mode otor enable helper is set, update that\ntree row item's value"
        n268 = event-data() -> ("NewVal"=w429:bool)  [unwired: 1 in]
        n269 = Unbundle("Motor") -> ("Value"=w428:dbl)  [unwired: 1 out]
        n270 = Select(t=w428, s=w429, f=0.0) -> (s? t:f=w426:dbl)
        n271 = call <vilib>:"NT Write Number.vi"("Numeric"=w426, "Name"=w425) -> ()  [unwired: 9 in, 1 out]
      }
      event "Test Slider": Value Change {
        # "When the test mode slider helper is set, update that\ntree row item's value"
        n272 = event-data() -> ("NewVal"=w432:dbl)  [unwired: 1 in]
        n273 = call <vilib>:"NT Write Number.vi"("Numeric"=w432, "Name"=w433) -> ()  [unwired: 9 in, 1 out]
      }
      event "On/Off": Value Change {
        # "When the test mode on/off helper value is set, update that\ntree row item's value"
        n274 = event-data() -> ("NewVal"=w437:bool)  [unwired: 1 in]
        n275 = Boolean To (0,1)(Boolean=w437) -> (0, 1=w436:i16)
        n276 = call <vilib>:"NT Write Number.vi"("Numeric"=w436, "Name"=w435) -> ()  [unwired: 9 in, 1 out]
      }
      event "Rev/Fwd": Value Change {
        # "When the test mode helper value for relays is set, update that\ntree row item's value"
        n277 = event-data() -> ("NewVal.Forward"=w445:bool, "NewVal.Reverse"=w444:bool)  [unwired: 1 in]
        n278 = Boolean To (0,1)(Boolean=w445) -> (0, 1=w441:i16)
        n279 = Boolean To (0,1)(Boolean=w444) -> (0, 1=w443:i16)
        n280 = Negate(x=w443) -> (-x=w442:i16)
        n281 = Add(x=w441, y=w442) -> (x+y=w440:i16)
        n282 = call <vilib>:"NT Write Number.vi"("Numeric"=w440, "Name"=w439) -> ()  [unwired: 9 in, 1 out]
      }
      event "Test Ring": Value Change {
        # "When a test mode helper value is selected from the ring,\nset the tree item's variable to the string value"
        n283 = event-data() -> ("NewVal"=w449:u16)  [unwired: 1 in]
        n284 = property on="Test Ring" class="Ring (strict)"() -> ("Strings []"=w450:string[])  [unwired: 2 in, 2 out]
        n285 = Index Array(array=w450, index=w449) -> (element=w448:string)
        n286 = call <vilib>:"NT Write String.vi"("String"=w448, "Name"=w447) -> ()  [unwired: 9 in, 1 out]
      }
      event "Rec Mode": Value Change {
        # "Update globals for recording mode and path to read log from.\nClear when logging and let NetworkTables set path for vision to\nuse."
        n287 = event-data() -> ("NewVal"=w461:enum32{"Stop", "Record", "Playback"})  [unwired: 1 in]
        n288 = global write "WPI_DashboardLogging Global.vi" "Logging Filename"(path "") -> ()
        n289 = global write "WPI_DashboardLogging Global.vi" "Recording"(w461) -> ()
        n290 = case shown="\"Playback\"" w461 {
          tunnel: w460 -> [_ w463 w472]
          tunnel: [_ _ w471] -> w458
          tunnel: [_ _ w470] -> _
          tunnel: w456 -> [_ _ w468]
          tunnel: cluster{i32, i32} {-250, 170} -> [_ _ w467]
          tunnel: [_ _ T22 {"Image Size"=TRUE, "Image Type"=TRUE, "Pixel Value"=TRUE, "ROI Information"=TRUE, "Zoom Factor"=FALSE} ("Image Information Shown:All Elements")] -> w451
          tunnel: [_ _ TRUE ("Zoom Factor")] -> w452
          tunnel: w454 -> [_ _ w464]
          frame Default {
          }
          frame "Stop", "Record" {
            # "Place Window too"
            n291 = invoke class="VI" method="FP.Close"(reference=w463) -> (reference out=w462:refnum<vi>)  [unwired: 2 in, 2 out]
            n292 = invoke class="VI" method="Abort VI"(reference=w462) -> ()  [unwired: 2 in, 3 out]
          }
          frame "Playback" {
            n293 = call "Open Playback Panel.vi"("Offset"=w467, "DB VI Ref"=w468, "Playback in"=w472) -> ("Playback out"=w469:refnum<vi>)  [unwired: 8 in]
            n294 = register-events(w469, w464) -> (reference out=w471:refnum<event-registration>, error out=w470:errorcluster)  [unwired: 2 in]
          }
        }
        n295 = property on="Camera Image Right" class="ImageControl"("Image Information Shown"=w451, "Image Information Visible"=w452) -> ()  [unwired: 2 in, 2 out]
        n296 = property on="Camera Image" class="ImageControl"("Image Information Shown"=w451, "Image Information Visible"=w452) -> ()  [unwired: 2 in, 2 out]
        n297 = call <vilib>:"WPI_DashboardNT Log FieldName Cache.vi"("Operation"=enum16{"Lookup/Add", "Index", "Clear"}."Clear") -> ()  [unwired: 8 in, 3 out]
      }
      event Panel Close {
        w474 = enum32{"Stop", "Record", "Playback"}."Stop" ("Rec Mode")
        # "Playback window has been closed, abort"
        n298 = event-data() -> ()  [unwired: 1 in, 4 out]
        n299 = local write "Rec Mode"(w474) -> ()
        n300 = global write "WPI_DashboardLogging Global.vi" "Recording"(w474) -> ()
      }
      event Panel Close {
        # "Abort playback window and ourself"
        n301 = event-data() -> ()  [unwired: 1 in, 4 out]
        n302 = invoke class="VI" method="FP.Close"(reference=w478) -> (reference out=w477:refnum<vi>)  [unwired: 2 in, 2 out]
        n303 = invoke class="VI" method="Abort VI"(reference=w477) -> (error out=w476:errorcluster)  [unwired: 2 in, 2 out]
        n304 = invoke class="VI" method="Abort VI"(error in=w476) -> ()  [unwired: 2 in, 3 out]
      }
      event User Event {
        n305 = event-data() -> ("IDs"=w485:cluster{"RPC field ID":u16, "Unique ID":u16}, "String"=w484:string)  [unwired: 1 in]
        n306 = Bundle("IDs"=w485, "String"=w484) -> (w483:T9)  [unwired: 1 in]
        n307 = call <vilib>:"Retrieve RPC Response.vi"("RPC Response"=w483) -> ("Output"=w481:string[][])  [unwired: 10 in]
        n308 = Build Array (concatenate)(w479, w481) -> (w480:string[][])
        n309 = local write "Command Params"(w480) -> ()
        n310 = local write "Cmd Status"("" ("Cmd Status")) -> ()
      }
      event "Tree": Double Click {
        n311 = event-data() -> ("PlatMods"=w491:T25, "Tag"=w488:string)  [unwired: 1 in]
        n312 = Unbundle(w491) -> ("Shift"=w490:bool)  [unwired: 4 out]
        n313 = String Subset(string=w488, length (rest)=1 ("length (rest)")) -> (substring=w487:string)  [unwired: 1 in]
        n314 = Not(x=w490) -> (.not. x?=w489:bool)
        n315 = case shown="\"/\"" w487 {
          tunnel: w488 -> [_ w494]
          tunnel: w489 -> [_ w493]
          frame Default {
          }
          frame "/" {
            n316 = call <vilib>:"NT Update Persistence.vi"("Persistence"=w493, "Name"=w494) -> ()  [unwired: 9 in, 1 out]
          }
        }
      }
    }
  }
  n317 = while {
    tunnel: w65 -> [w496]
    i -> [w499]
    stop <- FALSE stop-if-true
    n318 = Wait (ms)(milliseconds to wait=u32 100) -> ()  [unwired: 1 out]
    n319 = case shown="\"Playback\"" "Rec Mode" {
      tunnel: w499 -> [_ _ w514]
      tunnel: [u32 2829099 ("Base Color") u32 11141120 ("Target Color") w503] -> w495
      frame "Stop", Default {
        # "Reset the color, extra updates don't cost much"
      }
      frame "Record" {
      }
      frame "Playback" {
        # "Playback"
        n320 = Quotient & Remainder(x=w514, y=u32 50 ("milliseconds to wait")) -> (x-y*floor(x/y)=w510:u32)  [unwired: 1 out]
        n321 = Divide(x=w510, y=u32 50 ("milliseconds to wait")) -> (x/y=w507:dbl)
        n322 = Multiply(x=6.283185307179586, y=w507) -> (x*y=w512:dbl)
        n323 = Sine(x=w512) -> (sin(x)=w511:dbl)
        n324 = Absolute Value(x=w511) -> (abs(x)=w504:dbl)
        n325 = call "Interpolate RGB Color.vi"("Proportion"=w504, "Target Color"=u32 30976, "Base Color"=u32 2829099) -> ("Result Color"=w503:u32)  [unwired: 8 in]
      }
    }
    n326 = property class="Pane"(reference=w496, "PaneColor"=w495) -> ()  [unwired: 1 in, 2 out]
  }
  n327 = local write "Dashboard Tab"(T2."Drive" ("Dashboard Tab")) -> ()
  n328 = property on="On/Off" class="Bool (strict)"("Visible"=w36) -> ()  [unwired: 2 in, 2 out]
  n329 = property on="Motor" class="Clust (strict)"("Visible"=w36) -> ()  [unwired: 2 in, 2 out]
  n330 = property on="Progress" class="Clust (strict)"("Visible"=w36) -> ()  [unwired: 2 in, 2 out]
  n331 = property on="Test Ring" class="Ring (strict)"("Visible"=w36) -> ()  [unwired: 2 in, 2 out]
  n332 = property on="Rev/Fwd" class="Clust (strict)"("Visible"=w36) -> ()  [unwired: 2 in, 2 out]
  n333 = while {
    tunnel: u16 1741 ("timeout ms (25000)") -> [w516]
    stop <- FALSE stop-if-true
    n334 = TCP Create Listener(10:w516) -> (0:w515:errorcluster, 3:w517:refnum<k5>)  [unwired: 4 in, 1 out]
    n335 = case shown="No Error" w515 {
      selector: w515 -> [w519 _]
      tunnel: w517 -> [w520 _]
      frame No Error {
        n336 = while {
          tunnel: w520 -> [w523]
          tunnel: w519 -> [w522]
          stop <- FALSE stop-if-true
          n337 = TCP Wait On Listener(8:w522, 11:w523) -> (0:w524:errorcluster, 4:w525:refnum<k5>)  [unwired: 2 in, 3 out]
          n338 = local write "TCP"(w525) -> ()
          n339 = case shown="No Error" w524 {
            frame No Error {
            }
            frame Error {
              n340 = Wait (ms)(milliseconds to wait=u32 1000) -> ()  [unwired: 1 out]
            }
          }
        }
      }
      frame Error {
        n341 = Wait (ms)(milliseconds to wait=u32 1000) -> ()  [unwired: 1 out]
      }
    }
  }
  n342 = local write "Command Selection"(u16 0 ("milliseconds to wait")) -> ()
  n343 = local write "Command Params"(string[][] [] ("Command Params")) -> ()
  n344 = global write "WPI_DashboardLogging Global.vi" "Recording"(w59) -> ()
  n345 = local write "Rec Mode"(w59) -> ()
  n346 = call <vilib>:"NT Write String.vi"("String"="Select Auto", "Name"="Auto Selector") -> ()  [unwired: 9 in, 1 out]
